vi "Borders.vi"(8 "error in":errorcluster, 10 "Write/Read Cell":T1={"Cell Range"="", "Data 2D"=[], "Select Sheet"="", "1 Data"="", "Data 1D"=[], "Font col"=0, "Bold"=TRUE, "Font Size"=18, "Inside lines"=FALSE}, 11 "_Worksheet 2":refnum<k7>) -> (0 "error out":errorcluster, 3 "_Worksheet":refnum<k7>)   [LabVIEW 2017]
uses:
  controls/read.write.ctl
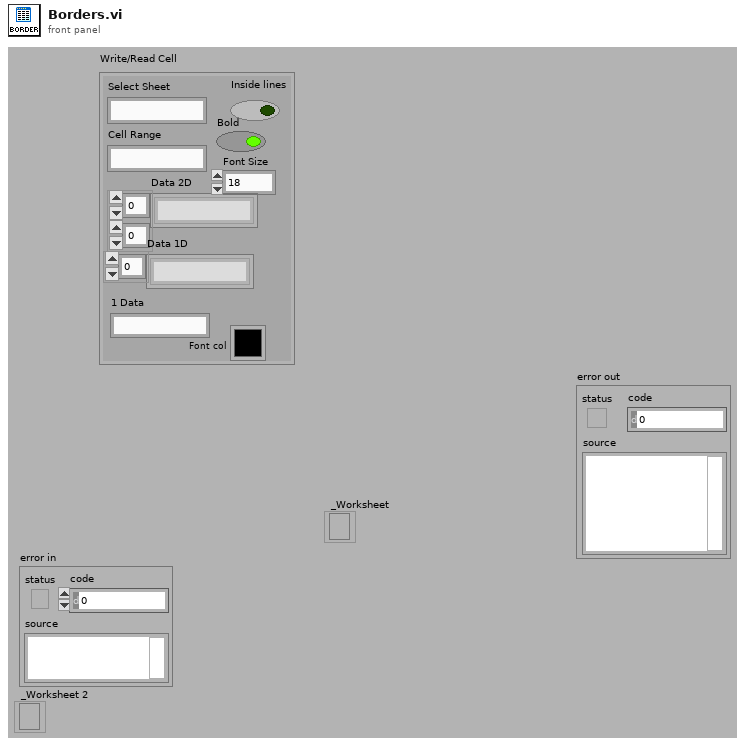
[diagram p1: front panel]
types:
  T1 = typedef "read.write.ctl" = cluster{"Cell Range":string, "Data 2D":string[][], "Select Sheet":string, "1 Data":string, "Data 1D":string[], "Font col":u32, "Bold":bool, "Font Size":i32, "Inside lines":bool}
  T2 = enum16{"xlNone", "xlContinuous", "xlDot", "xlDashDot", "xlDash", "xlDashDotDot", "xlSlantDashDot", "xlDouble"}
  T3 = enum16{"xlNone", "xlThin", "xlHairline", "xlMedium", "xlThick"}
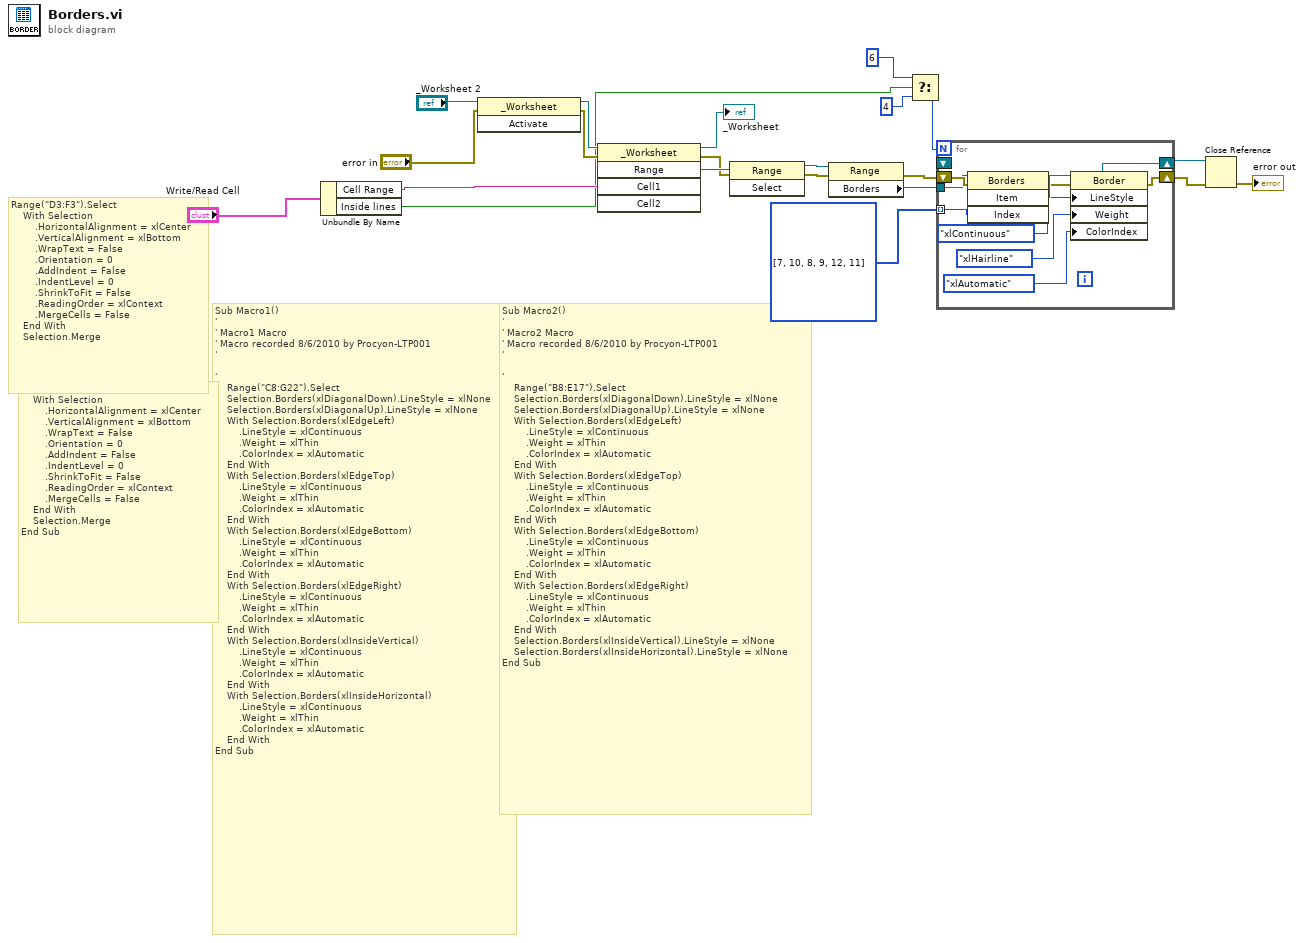
[diagram p0: block diagram]
diagram:
  w6 = i32[] [7, 10, 8, 9, 12, 11] items=["xlInsideHorizontal"=12, "xlInsideVertical"=11, "xlDiagonalDown"=5, "xlDiagonalUp"=6, "xlEdgeBottom"=9, "xlEdgeLeft"=7, "xlEdgeRight"=10, "xlEdgeTop"=8]
  # "Sub Macro2()\n'\n' Macro2 Macro\n' Macro recorded 8/6/2010 by Procyon-LTP001\n'\n\n'\n    Range(\"B8:E17\").Select\n    Selection.Borders(xlDiagonalDown).LineStyle = xlNone\n    Selection.Borders(xlDiagonalUp).LineStyle = xlNone\n    With Selection.Borders(xlEdgeLeft)\n        .LineStyle = xlContinuous\n        .Weight = xlThin\n        .ColorIndex = xlAutomatic\n    End With\n    With Selection.Borders(xlEdgeTop)\n        .LineStyle = xlContinuous\n        .Weight = xlThin\n        .ColorIndex = xlAutomatic\n    End With\n    With Selection.Borders(xlEdgeBottom)\n        .LineStyle = xlContinuous\n        .Weight = xlThin\n        .ColorIndex = xlAutomatic\n    End With\n    With Selection.Borders(xlEdgeRight)\n        .LineStyle = xlContinuous\n        .Weight = xlThin\n        .ColorIndex = xlAutomatic\n    End With\n    Selection.Borders(xlInsideVertical).LineStyle = xlNone\n    Selection.Borders(xlInsideHorizontal).LineStyle = xlNone\nEnd Sub"
  # "Sub Macro1()\n'\n' Macro1 Macro\n' Macro recorded 8/6/2010 by Procyon-LTP001\n'\n\n'\n    Range(\"C8:G22\").Select\n    Selection.Borders(xlDiagonalDown).LineStyle = xlNone\n    Selection.Borders(xlDiagonalUp).LineStyle = xlNone\n    With Selection.Borders(xlEdgeLeft)\n        .LineStyle = xlContinuous\n        .Weight = xlThin\n        .ColorIndex = xlAutomatic\n    End With\n    With Selection.Borders(xlEdgeTop)\n        .LineStyle = xlContinuous\n        .Weight = xlThin\n        .ColorIndex = xlAutomatic\n    End With\n    With Selection.Borders(xlEdgeBottom)\n        .LineStyle = xlContinuous\n        .Weight = xlThin\n        .ColorIndex = xlAutomatic\n    End With\n    With Selection.Borders(xlEdgeRight)\n        .LineStyle = xlContinuous\n        .Weight = xlThin\n        .ColorIndex = xlAutomatic\n    End With\n    With Selection.Borders(xlInsideVertical)\n        .LineStyle = xlContinuous\n        .Weight = xlThin\n        .ColorIndex = xlAutomatic\n    End With\n    With Selection.Borders(xlInsideHorizontal)\n        .LineStyle = xlContinuous\n        .Weight = xlThin\n        .ColorIndex = xlAutomatic\n    End With\nEnd Sub"
  # "Range(\"A3:F3\").Select\n    With Selection\n        .HorizontalAlignment = xlCenter\n        .VerticalAlignment = xlBottom\n        .WrapText = False\n        .Orientation = 0\n        .AddIndent = False\n        .IndentLevel = 0\n        .ShrinkToFit = False\n        .ReadingOrder = xlContext\n        .MergeCells = False\n    End With\n    Selection.Merge\nEnd Sub"
  # "Range(\"D3:F3\").Select\n    With Selection\n        .HorizontalAlignment = xlCenter\n        .VerticalAlignment = xlBottom\n        .WrapText = False\n        .Orientation = 0\n        .AddIndent = False\n        .IndentLevel = 0\n        .ShrinkToFit = False\n        .ReadingOrder = xlContext\n        .MergeCells = False\n    End With\n    Selection.Merge"
  n1 = Unbundle By Name("Write/Read Cell") -> ("Cell Range"=w12:string, "Inside lines"=w1:bool)
  n2 = invoke class="_Worksheet" method="Activate"(reference="_Worksheet 2", error in="error in") -> (reference out=w15:refnum<k7>, error out=w13:errorcluster)  [unwired: 1 in, 1 out]
  n3 = invoke class="_Worksheet" method="Range"(reference=w15, error in=w13, "Cell1"=w12) -> (reference out=→"_Worksheet":refnum<k7>, error out=w20:errorcluster, "Range"=w21:refnum<k7>)  [unwired: 2 in, 2 out]
  n4 = invoke class="Range" method="Select"(reference=w21, error in=w20) -> (reference out=w19:refnum<k7>, error out=w18:errorcluster)  [unwired: 1 in, 1 out]
  n5 = property class="Range"(reference=w19, error in=w18) -> (error out=w11:errorcluster, "Borders"=w10:refnum<k7>)  [unwired: 1 out]
  n6 = Select(t=6, s=w1, f=4) -> (s? t:f=w3:i32)
  n7 = for {
    N: w3 -> [_]
    tunnel: w10 -> [w30]
    tunnel: w6 -> [w28] mode=indexing
    shift-right: [w24] -> w8
    shift-left: w11 -> [w31]
    shift-right: [w22] -> w9
    shift-left: _ -> [_]
    n8 = invoke class="Borders" method="Item"(reference=w30, error in=w31, "Index"=w28) -> (reference out=w22:refnum<k7>, error out=w25:errorcluster, "Item"=w29:refnum<k7>)  [unwired: 1 in, 1 out]
    n9 = property class="Border"(reference=w29, error in=w25, "LineStyle"=T2."xlContinuous", "Weight"=T3."xlHairline", "ColorIndex"=enum16{"xlAutomatic"}."xlAutomatic") -> (error out=w24:errorcluster)  [unwired: 1 out]
  }
  n10 = Close Reference(reference=w9, error in (no error)=w8) -> (error out=→"error out":errorcluster)
